vi "LibraryRefProbe.vi"(11 "Library Refnum":refnum<vi>) -> (2 "Display string":string, 3 "Stop?":bool)   [LabVIEW 2020]
doc: "Displays the VI name, the VI path, and the hex value of the reference. You can use this probe to set a breakpoint if the value is an invalid refnum."
uses:
  <vilib>/Utility/error.llb/DialogTypeEnum.ctl
panel:
  in  "application instance":string="Application instance"
  in  "error source":string="Library Refnum Probe"
  in  "lib path":string="Library path"
  in  "lib name":string="Library name"
  in  "Pause if Not a Refnum":bool
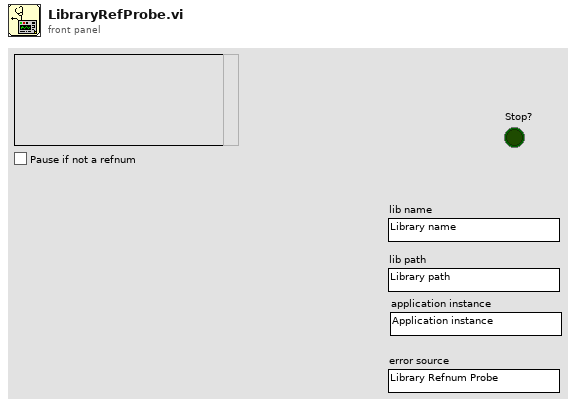
[diagram p1: front panel]
types:
  T1 = typedef "DialogTypeEnum.ctl" = enum16{"no dialog", "OK message", "continue or stop message", "auto error handling dialog", "OK message + warnings", "continue/stop + warnings"}
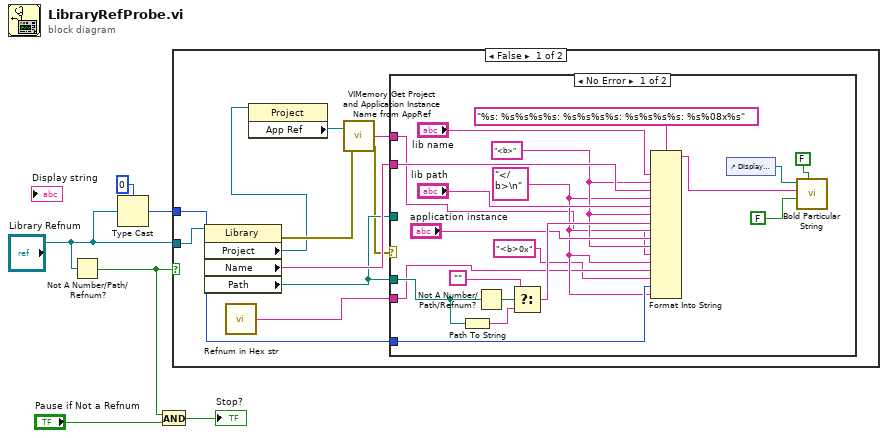
[diagram p0: block diagram]
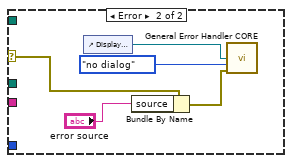
[diagram p2: hidden frame]
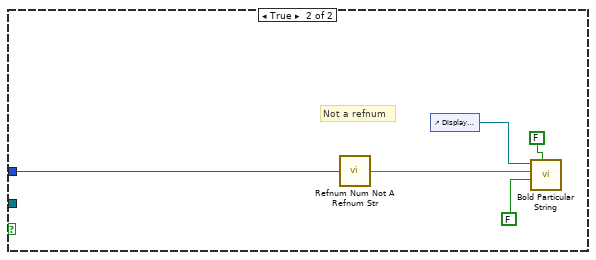
[diagram p3: hidden frame]
diagram:
  n1 = Not A Number/Path/Refnum?(number/path/refnum="Library Refnum") -> (NaN/Path/Refnum?=w4:bool)
  n2 = Type Cast(type=u32 0, x="Library Refnum") -> (*(type *) &x=w1:u32)
  n3 = And(x=w4, y="Pause if Not a Refnum") -> (x .and. y?=→"Stop?":bool)
  n4 = case shown="False" w4 {
    tunnel: "Library Refnum" -> [w9 _]
    tunnel: w1 -> [w14 w43]
    frame False {
      n5 = property class="Library"(reference=w9) -> (error out=w11:errorcluster, "Project"=w7:refnum<vi>, "Name"=w16:string, "Path"=w15:path)  [unwired: 1 in, 1 out]
      n6 = call <vilib>:"Refnum in Hex str.vi"() -> ("refnum in hex"=w13:string)
      n7 = property class="Project"(reference=w7) -> ("App Ref"=w8:refnum<vi>)  [unwired: 1 in, 2 out]
      n8 = call <vilib>:"VIMemory Get Project and Application Instance Name from AppRef.vi"("app reference"=w8, "error in (no error)"=w11) -> ("Project and Application Instance Name"=w12:string, "error out"=w10:errorcluster)  [unwired: 1 out]
      n9 = case shown="No Error" w10 {
        selector: w10 -> [_ w38]
        tunnel: w14 -> [w22 _]
        tunnel: w13 -> [w18 _]
        tunnel: w15 -> [_ _]
        tunnel: w16 -> [w26 _]
        tunnel: w15 -> [w31 _]
        tunnel: w12 -> [w19 _]
        frame No Error {
          w20 = "</b>\n"
          w21 = "<b>"
          n10 = Path To String(path=w31) -> (string=w33:string)
          n11 = Not A Number/Path/Refnum?(number/path/refnum=w31) -> (NaN/Path/Refnum?=w34:bool)
          n12 = Select(t="", s=w34, f=w33) -> (s? t:f=w28:string)
          n13 = Format Into String(format string="%s: %s%s%s%s: %s%s%s%s: %s%s%s%s: %s%08x%s", "lib name", w21, w26, w20, "lib path", w21, w28, w20, "application instance", w21, w19, w20, w18, "<b>0x", w22, w20) -> (resulting string=w29:string)  [unwired: 2 in, 1 out]
          n14 = control-ref of="Display string"() -> (w36:refnum<vi>)
          n15 = call <vilib>:"Bold Particular String.vi"("Always Refresh? (TRUE)"=FALSE ("Always Refresh? (FALSE)"), "resize string? (TRUE)"=FALSE ("resize string?"), "text to display"=w29, "string refnum"=w36) -> ()  [unwired: 6 in, 2 out]
        }
        frame Error {
          n16 = control-ref of="Display string"() -> (w37:refnum<vi>)
          n17 = Bundle By Name(cluster=w38, "source"="error source") -> (w40:errorcluster)
          n18 = call <vilib>:"General Error Handler CORE.vi"("String to Format (not a refnum)"=w37, "type of dialog (OK msg:1)"=DialogTypeEnum."no dialog", "error in (no error)"=w40) -> ()  [unwired: 7 in, 6 out]
        }
      }
    }
    frame True {
      # "Not a refnum"
      n19 = call <vilib>:"Refnum Num Not A Refnum Str.vi"("Numeric"=w43) -> ("text to display"=w42:string)
      n20 = control-ref of="Display string"() -> (w45:refnum<vi>)
      n21 = call <vilib>:"Bold Particular String.vi"("Always Refresh? (TRUE)"=FALSE ("Always Refresh? (FALSE)"), "resize string? (TRUE)"=FALSE, "text to display"=w42, "string refnum"=w45) -> ()  [unwired: 6 in, 2 out]
    }
  }
